vi "TDMS Advanced Finite Asynchronous Read.vi"() -> ()   [LabVIEW 2023]
doc: "This example demonstrates how to read data asynchronously from a .tdms file using the Advanced TDMS VIs and functions. Users can specify a finite number of available buffers to read."
panel:
  out "Waveform Graph":u32[](graph)
  # "Overview: Demonstrates the use of the Advanced TDMS functions to read a .tdms file asynchronously. Users can specify a finite number of available buffers to read.\nInstructions:\n1. Make sure you have already run TDMS Advanced Asynchronous Write.vi.\n2. Run this VI.\n3. Delete the TDMS file (located at [LabVIEW Data]\\Example TDMS Advanced Asynchronous Write.tdms) when you are done."
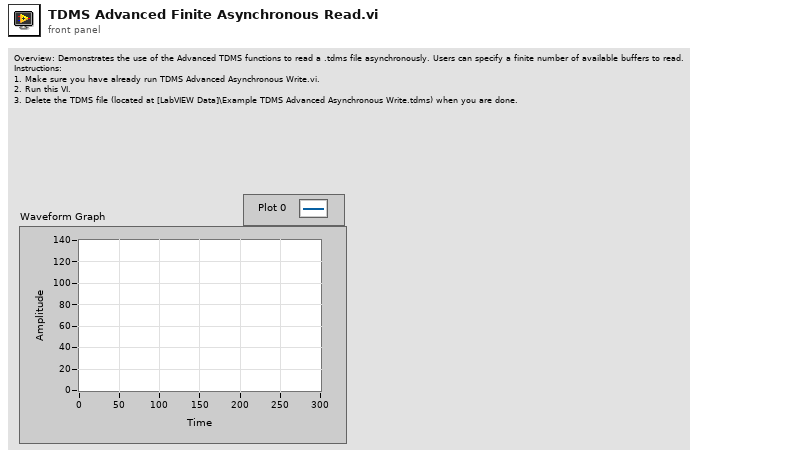
[diagram p1: front panel]
types:
  T1 = enum16{"open", "open or create", "create or replace", "create", "open (read-only)"}
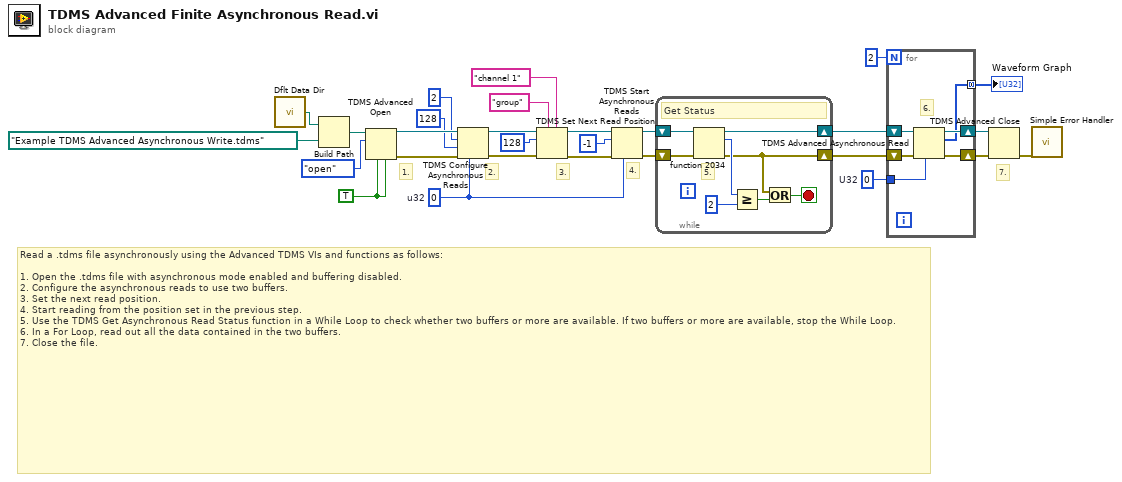
[diagram p0: block diagram]
diagram:
  w3 = u32 0  # U32
  w2 = u32 0  # u32
  w24 = TRUE ("enable asynchronous? (T)")
  # "3."
  # "4."
  # "2."
  # "Read a .tdms file asynchronously using the Advanced TDMS VIs and functions as follows:\n\n1. Open the .tdms file with asynchronous mode enabled and buffering disabled.\n2. Configure the asynchronous reads to use two buffers.\n3. Set the next read position.\n4. Start reading from the position set in the previous step.\n5. Use the TDMS Get Asynchronous Read Status function in a While Loop to check whether two buffers or more are available. If two buffers or more are available, stop the While Loop.\n6. In a For Loop, read out all the data contained in the two buffers.\n7. Close the file."
  # "1."
  # "7."
  n1 = call <vilib>:"Dflt Data Dir.vi"() -> ("App:Default Data Directory"=w25:path)
  n2 = Build Path(base path=w25, name or relative path=path "Example TDMS Advanced Asynchronous Write.tdms") -> (appended path=w27:path)
  n3 = TDMS Advanced Open(4:w24, 6:w24, 10:T1."open" ("operation (0:open)"), 11:w27) -> (0:w22:errorcluster, 3:w23:refnum<k34>)  [unwired: 1 in, 1 out]
  n4 = TDMS Configure Asynchronous Reads(6:w2, 8:w22, 9:u32 128 ("buffer size"), 10:u32 2 ("number of buffers (4)"), 11:w23) -> (0:w16:errorcluster, 3:w15:refnum<k34>)  [unwired: 1 in]
  n5 = TDMS Set Next Read Position(5:"channel 1" ("channel name in"), 7:"group" ("group name in"), 8:w16, 10:i64 128 ("offset (0)"), 11:w15) -> (0:w11:errorcluster, 3:w10:refnum<k34>)  [unwired: 1 in]
  n6 = TDMS Start Asynchronous Reads(6:w2, 8:w11, 10:i64 -1 ("total count (-1)"), 11:w10) -> (0:w17:errorcluster, 3:w18:refnum<k34>)
  n7 = while {
    shift-right: [w36] -> w7
    shift-left: w18 -> [w34]
    shift-right: [w29] -> w6
    shift-left: w17 -> [w33]
    stop <- w30 stop-if-true
    # "5."
    # "Get Status"
    n8 = fn#2034(8:w33, 11:w34) -> (0:w29:errorcluster, 2:w32:u32, 3:w36:refnum<k34>)  [unwired: 1 out]
    n9 = Greater Or Equal?(x=w32, y=2) -> (x >= y?=w31:bool)
    n10 = Or(x=w29, y=w31) -> (x .or. y?=w30:bool)
  }
  n11 = for {
    N: 2 -> [_]
    shift-right: [w42] -> w9
    shift-left: w6 -> [w39]
    shift-right: [w41] -> w8
    shift-left: w7 -> [w40]
    tunnel: w3 -> [w38]
    tunnel: [w37] -> w1 mode=concatenating
    # "6."
    n12 = TDMS Advanced Asynchronous Read(6:w38, 8:w39, 11:w40) -> (0:w42:errorcluster, 2:w37:u32[], 3:w41:refnum<k34>)  [unwired: 1 out]
  }
  "Waveform Graph" <- w1
  n13 = TDMS Advanced Close(8:w9, 11:w8) -> (0:w4:errorcluster)  [unwired: 2 in, 1 out]
  n14 = call <vilib>:"Simple Error Handler.vi"("error in (no error)"=w4) -> ()  [unwired: 4 in, 5 out]
